vi "MAX_ASCII.vi"() -> ()   [LabVIEW 2017]
uses:
  <vilib>/Instr/_visa.llb/VISA Configure Serial Port (Instr).vi
panel:
  in  "flow control":u16(ring) items=["None", "XON/XOFF", "RTS/CTS", "XON/XOFF & RTS/CTS", "DTR/DSR", "XON/XOFF & DTR/DSR"]
  in  "parity":enum16{"None", "Odd", "Even", "Mark", "Space"}(ring)
  in  "data bits":u16=8 min=5 max=8 step=1
  in  "baud rate":u32=9600
  in  "stop bits":u16(ring)=10 items=["1.0"=10, "1.5"=15, "2.0"=20]
  out "concatenated string":string
  out "Table of data":string[][](table)
  in  "Start Reading":bool
  in  "Stop Simulation":bool
  in  "Serial Port":refnum<visa-resource-name>
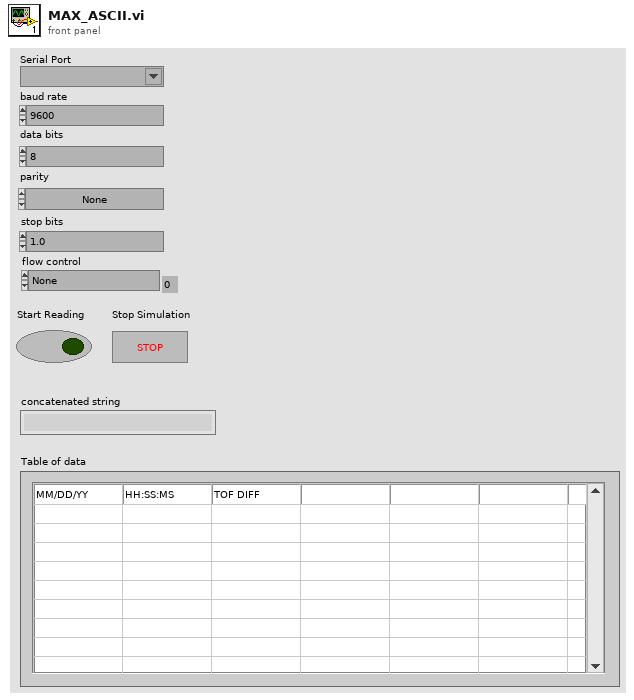
[diagram p1: front panel]
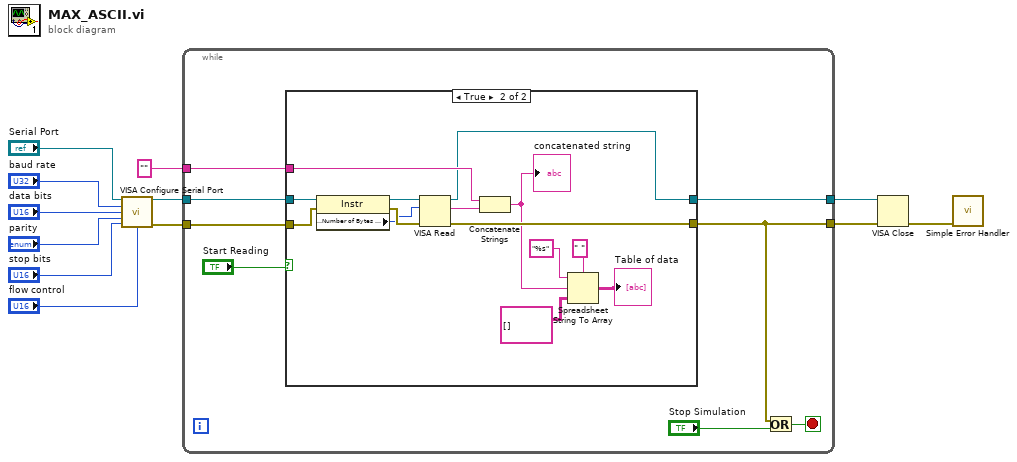
[diagram p0: block diagram]
diagram:
  n1 = call-poly "VISA Configure Serial Port"("VISA resource name"="Serial Port", "baud rate (9600)"="baud rate", "data bits (8)"="data bits", "parity (0:none)"="parity", "stop bits (10: 1 bit)"="stop bits", "flow control (0:none)"="flow control") -> ("VISA resource name out"=w8:refnum<visa-resource-name>, "error out"=w12:errorcluster)  [unwired: 8 in]
  n2 = while {
    tunnel: w12 -> [w20]
    tunnel: [w16] -> w11
    tunnel: [w15] -> w10
    tunnel: w8 -> [w13]
    tunnel: "" ("string") -> [w14]
    stop <- w18 stop-if-true
    n3 = case shown="True" "Start Reading" {
      tunnel: w20 -> [w21 w35]
      tunnel: [w21 w36] -> w16
      tunnel: [w22 w29] -> w15
      tunnel: w14 -> [_ w30]
      tunnel: w13 -> [w22 w28]
      frame False {
      }
      frame True {
        n4 = property class="Instr"(reference=w28, error in=w35) -> (reference out=w33:refnum<visa-resource-name>, error out=w34:errorcluster, "Serial Settings:Number of Bytes at Serial Port"=w32:u32)
        n5 = VISA Read(VISA resource name=w33, byte count=w32, error in (no error)=w34) -> (VISA resource name out=w29:refnum<visa-resource-name>, read buffer=w31:string, error out=w36:errorcluster)  [unwired: 1 out]
        n6 = Concatenate Strings(w30, w31) -> (w27:string)
        "concatenated string" <- w27
        n7 = Spreadsheet String To Array(delimiter (Tab)=" ", format string="%s", spreadsheet string=w27, array type (2D Dbl)=string[][] [] ("Array")) -> (array=→"Table of data":string[][])
      }
    }
    n8 = Or(x=w16, y="Stop Simulation") -> (x .or. y?=w18:bool)
  }
  n9 = VISA Close(VISA resource name=w10, error in (no error)=w11) -> (error out=w7:errorcluster)
  n10 = call <vilib>:"Simple Error Handler.vi"("error in (no error)"=w7) -> ()  [unwired: 4 in, 5 out]
